vi "Get List of SBlocks in the Library.vi"() -> (0 "Subpanel Refs":refnum<vi>[](array[refnum]), 1 "List of Available SBlock Types":string[](array[string]))   [LabVIEW 2020, in "Run Utilities.lvlib"]
doc: "This VI searches the library for all children of the Schedule Block class and returns the list of available types. The type names are inferred from the sblock class name (should be of the format \"<type> SBlock.lvclass\")."
uses:
  Run Utilities.lvlib
  Schedule Block/Schedule Block.lvclass
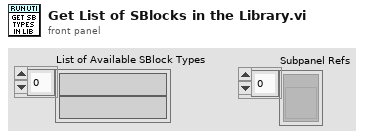
[diagram p1: front panel]
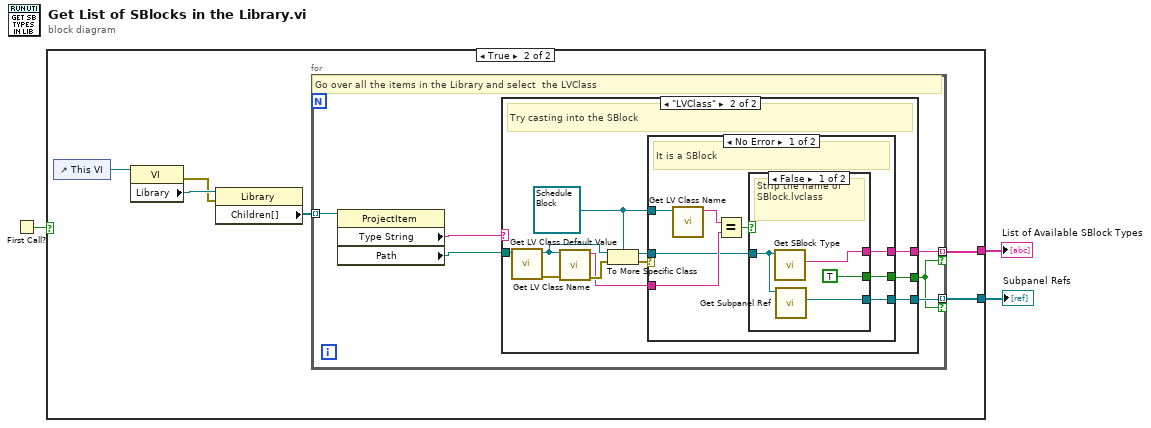
[diagram p0: block diagram]
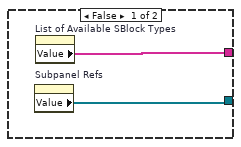
[diagram p2: hidden frame]
diagram:
  n1 = First Call?() -> (First Call?: T/F=w2:bool)
  n2 = case shown="True" w2 {
    tunnel: [w5 w7] -> w3
    tunnel: [w4 w6] -> w1
    frame False {
      n3 = property on="Subpanel Refs" class="Arr (strict)"() -> ("Value"=w4:refnum<vi>[])  [unwired: 2 in, 2 out]
      n4 = property on="List of Available SBlock Types" class="Arr (strict)"() -> ("Value"=w5:string[])  [unwired: 2 in, 2 out]
    }
    frame True {
      n5 = control-ref of="This VI"() -> (w11:refnum<vi>)
      n6 = property class="VI"(reference=w11) -> (error out=w9:errorcluster, "Library"=w10:refnum<vi>)  [unwired: 1 in, 1 out]
      n7 = property class="Library"(reference=w10, error in=w9) -> ("Children[]"=w8:refnum<vi>[])  [unwired: 2 out]
      n8 = for {
        tunnel: w8 -> [w17] mode=indexing
        tunnel: [w14] -> w7 mode=indexing if=w12
        tunnel: [w13] -> w6 mode=indexing if=w12
        # "Go over all the items in the Library and select  the LVClass"
        n9 = property class="ProjectItem"(reference=w17) -> ("Type String"=w16:string, "Path"=w15:path)  [unwired: 1 in, 2 out]
        n10 = case shown="\"LVClass\"" w16 {
          tunnel: w15 -> [_ w28]
          tunnel: [_ w24] -> w14
          tunnel: [_ w25] -> w12
          tunnel: [_ w18] -> w13
          frame Default {
          }
          frame "LVClass" {
            w26 = refnum<class "Schedule Block.lvclass"> refnum ("TALOS.lvlib:Run Utilities.lvlib:Schedule Block.lvclass")
            # "Try casting into the SBlock"
            n11 = call <vilib>:"Get LV Class Default Value.vi"("class path"=w28) -> ("error out"=w23:errorcluster, "object"=w21:refnum<class>)  [unwired: 9 in]
            n12 = call <vilib>:"Get LV Class Name.vi"("error in (no error)"=w23, "object"=w21) -> ("error out"=w22:errorcluster, "class name"=w20:string)  [unwired: 8 in]
            n13 = To More Specific Class(target class=w26, reference=w21, error in=w22) -> (specific class reference=w19:refnum<class "Schedule Block.lvclass">, error out=w27:errorcluster)
            n14 = case shown="No Error" w27 {
              tunnel: w26 -> [w36 _]
              tunnel: [w32 _] -> w25
              tunnel: [w33 _] -> w24
              tunnel: w20 -> [w31 _]
              tunnel: w19 -> [w30 _]
              tunnel: [w29 _] -> w18
              frame No Error {
                # "It is a SBlock"
                n15 = call <vilib>:"Get LV Class Name.vi"("object"=w36) -> ("class name"=w35:string)  [unwired: 9 in, 1 out]
                n16 = Equal?(x=w35, y=w31) -> (x = y?=w34:bool)
                n17 = case shown="False" w34 {
                  tunnel: [w39 _] -> w33
                  tunnel: [TRUE _] -> w32
                  tunnel: w30 -> [w38 _]
                  tunnel: [w37 _] -> w29
                  frame False {
                    # "Strip the name of SBlock.lvclass"
                    n18 = call-dynamic "Get SBlock Type.vi"("Schedule Block in"=w38) -> ("SBlock Type"=w39:string)  [unwired: 8 in, 2 out]
                    n19 = call-dynamic "Get Subpanel Ref.vi"("Schedule Block in"=w38) -> ("vi reference"=w37:refnum<vi>)  [unwired: 8 in, 2 out]
                  }
                  frame True {
                    # "Ignore the base class"
                  }
                }
              }
              frame Error {
                # "Not a SBlock, ignore"
              }
            }
          }
        }
      }
    }
  }
  "List of Available SBlock Types" <- w3
  "Subpanel Refs" <- w1
